vi "TestReadFromSF.vi"() -> ()   [LabVIEW 2009]
uses:
  <vilib>/Platform/TimedLoop/XDataNode/XDataNode.xnode
  <vilib>/Platform/TimedLoop/XDataNode/loadlvalarms.vi
  <vilib>/Platform/TimedLoop/XDataNode/timing_clust.ctl
  <vilib>/Platform/TimedLoop/XDataNode/nitl_modes.ctl
  <vilib>/Platform/TimedLoop/XDataNode/wakeup.ctl
  <vilib>/Platform/TimedLoop/XDataNode/XDNodeRunTimeDep.lvlib
panel:
  out "string":string
  in  "header size":i32
  in  "bytes to read":i32
  out "u2":sgl
  out "xa2":sgl
  out "u1":sgl
  out "x8":sgl
  out "x6":sgl
  out "x7":sgl
  out "x5":sgl
  out "xa1":sgl
  out "x3":sgl
  out "x4":sgl
  out "x1":sgl
  out "x2":sgl
  in  "Enable":bool
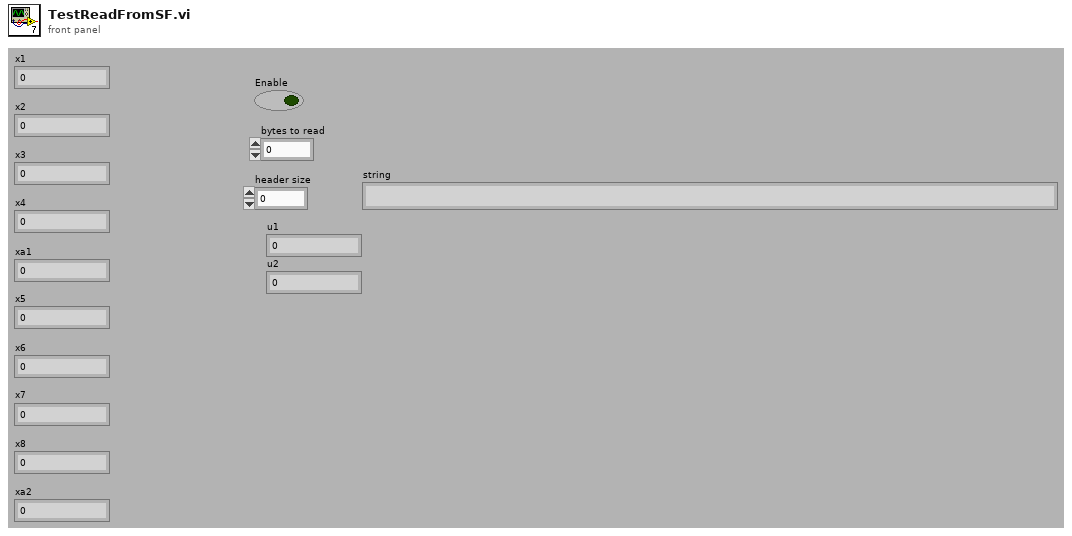
[diagram p1: front panel]
types:
  T1 = typedef "XDNodeRunTimeDep.lvlib/timing_clust.ctl" = cluster{"Expected End [f-1]":u64, "Actual End [f-1]":u64, "Finished Late? [f-1]":bool, "Expected End [i-1]":u64, "Actual End [i-1]":u64, "Finished Late? [i-1]":bool, "Expected Start [i]":u64, "Actual Start [i]":u64, "Expected Start [f]":u64, "Actual Start [f]":u64, "Source Name":string, "Structure Name":string, "Period":i64, "Deadline":i64, "Offset":i64, "Start":i64, "Priority":i32, "Timeout":i32, "Mode":T2, "Wakeup Reason":T3, "Error":errorcluster, "Source Type":string, "Secondary Source Type":string, "Global End Time":u64, "Global Start Time":u64, "Frame Duration":u64, "Iteration Duration":u64, "Assigned CPU":i32, "I/O Scan Engine Mode":u32}
  T2 = typedef "XDNodeRunTimeDep.lvlib/nitl_modes.ctl" = enum32{"No Change", "Process missed periods, maintain original phase", "Discard missed periods, maintain original phase", "Process missed periods, ignore original phase", "Discard missed periods, ignore original phase"}
  T3 = typedef "XDNodeRunTimeDep.lvlib/wakeup.ctl" = enum32{"Normal", "Aborted", "Asynchronous wakeup", "Timing source error", "Timed loop error", "Timeout"}
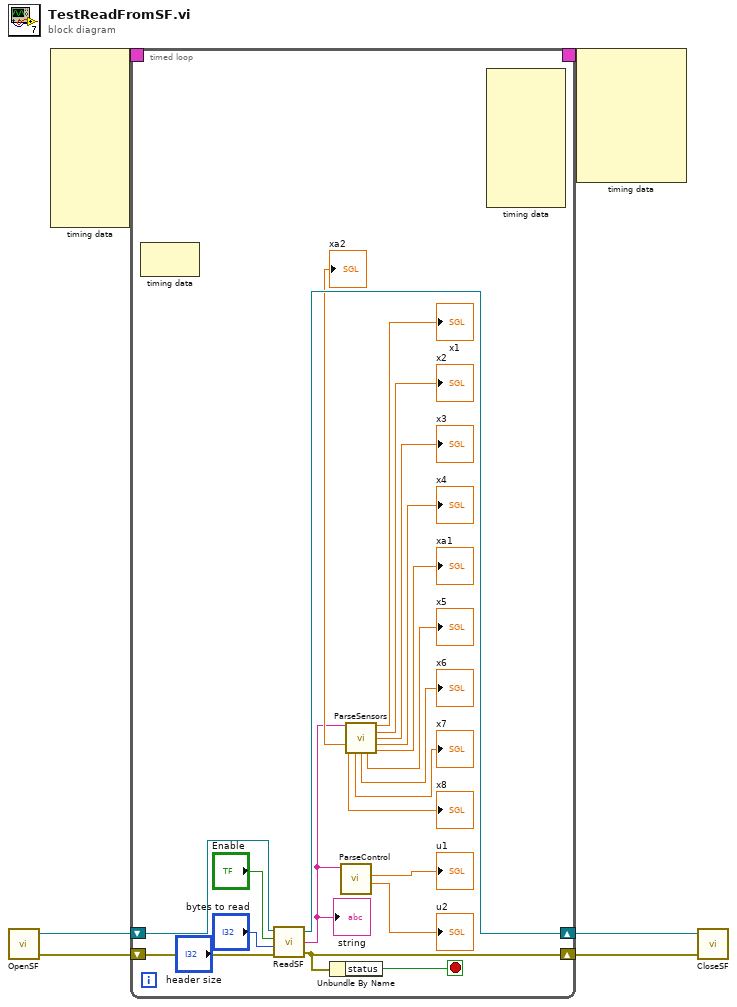
[diagram p0: block diagram]
diagram:
  n1 = call "OpenSF.vi"() -> ("error out"=w3:errorcluster, "connection ID"=w4:refnum<k5>)  [unwired: 1 out]
  n2 = node-c288() -> (w6:T1)  [unwired: 10 in]
  n3 = timed-loop {
    timing: w6 -> [_]
    timing-out: [_] -> w5
    shift-right: [w24] -> w2
    shift-left: w4 -> [w26]
    shift-right: [w25] -> w1
    shift-left: w3 -> [w8]
    stop <- w27 stop-if-true
    n4 = node-c288() -> ()  [unwired: 1 in, 1 out]
    n5 = call "ReadSF.vi"("connection ID in"=w26, "enabled"="Enable", "bytes to read"="bytes to read", "header size"="header size", "error in"=w8) -> ("connection ID out"=w24:refnum<k5>, "string"=w11:string, "error out"=w25:errorcluster)
    "string" <- w11
    n6 = Unbundle By Name(w25) -> ("status"=w27:bool)
    n7 = call "ParseControl.vi"("data out"=w11) -> ("u2"=→"u2":sgl, "u1"=→"u1":sgl)  [unwired: 4 in, 3 out]
    n8 = call "ParseSensors.vi"("data out"=w11) -> ("x1"=→"x1":sgl, "x2"=→"x2":sgl, "x3"=→"x3":sgl, "xa2"=→"xa2":sgl, "x4"=→"x4":sgl, "x8"=→"x8":sgl, "x7"=→"x7":sgl, "x6"=→"x6":sgl, "x5"=→"x5":sgl, "xa1"=→"xa1":sgl)  [unwired: 5 in]
    n9 = node-c288() -> ()  [unwired: 8 in, 1 out]
  }
  n10 = node-c288(w5) -> ()  [unwired: 7 out]
  n11 = call "CloseSF.vi"("error out"=w1, "connection ID"=w2) -> ()  [unwired: 1 in]
